vi "7.3-LoadFromFileEventHandler.vi"(0 "MissionDefFile":picture) -> (1 "Number of Waypoints Read":i32, 2 "MDF Out":T1 {"Latitude (waypoint)" format="%#_8g"; "Longitude  (waypoint)" format="%#_8g"}, 3 "new picture":picture)   [LabVIEW 2010]
uses:
  6-OCU Neurons/MDF Array LatLong.ctl
  6-OCU Neurons/MDF LatLong.ctl
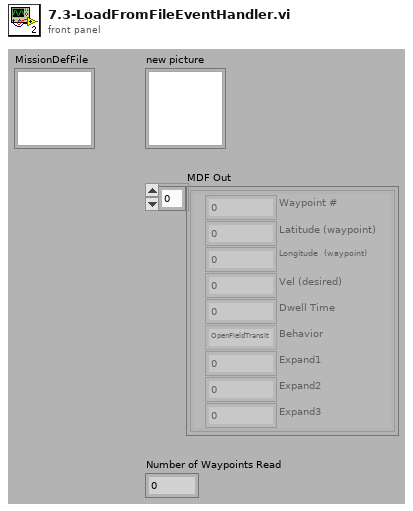
[diagram p1: front panel]
types:
  T1 = typedef "MDF Array LatLong.ctl" = T2[]
  T2 = typedef "MDF LatLong.ctl" = cluster{"Waypoint #":dbl, "Latitude (waypoint)":ext, "Longitude  (waypoint)":ext, "Vel (desired)":dbl, "Dwell Time":dbl, "Behavior":enum16{"OpenFieldTransit", "WallFollow", "LaneFollow", "ManualMode"}, "Expand1":dbl, "Expand2":dbl, "Expand3":dbl}
  T3 = cluster{"Width":u16, "Style":enum32{"Solid", "Dash", "Dot", "DashDot", "DashDotDot"}}
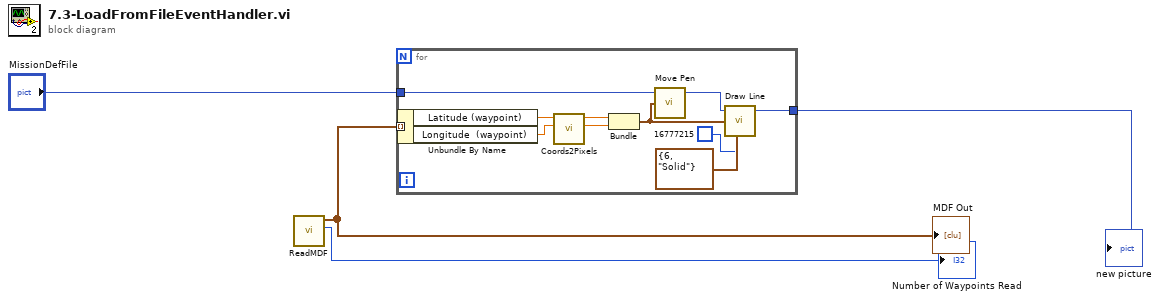
[diagram p0: block diagram]
diagram:
  n1 = call "ReadMDF.vi"() -> ("Number of Waypoints Read"=→"Number of Waypoints Read":i32, "MDF Out"=w4:T1)  [unwired: 9 in]
  "MDF Out" <- w4
  n2 = for {
    tunnel: "MissionDefFile" -> [w15]
    tunnel: [w13] -> w3
    tunnel: w4 -> [w7] mode=indexing
    n3 = Unbundle By Name(w7) -> ("Latitude (waypoint)"=w6:ext, "Longitude  (waypoint)"=w5:ext)
    n4 = call "Coords2Pixels.vi"("Latitude"=w5, "Longitude"=w6) -> ("Y"=w8:ext, "X"=w9:ext)  [unwired: 8 in]
    n5 = Bundle("X"=w9, "Y"=w8) -> (w12:cluster{"X":ext, "Y":ext})  [unwired: 1 in]
    n6 = call <vilib>:"Move Pen.vi"("new position"=w12, "picture"=w15) -> ("new picture"=w14:picture)  [unwired: 3 in]
    n7 = call <vilib>:"Draw Line.vi"("picture"=w14, "end point"=w12, "color(black)"=u32 16777215, "pen"=T3 {"Width"=6, "Style"=enum."Solid"}) -> ("new picture"=w13:picture)  [unwired: 5 in]
  }
  "new picture" <- w3
